vi "3.2 resolve.vi"() -> ()   [LabVIEW 2017]
panel:
  out "Numeric":i32
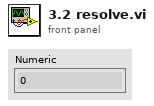
[diagram p1: front panel]
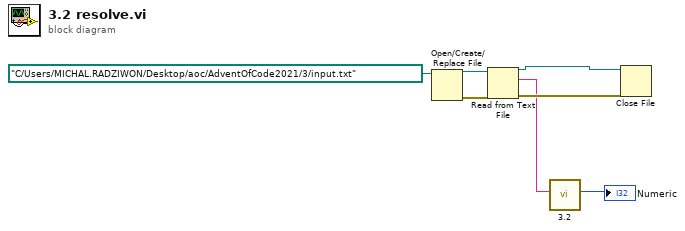
[diagram p0: block diagram]
diagram:
  n1 = Open/Create/Replace File(file path (use dialog)=path "C:/Users/MICHAL.RADZIWON/Desktop/aoc/AdventOfCode2021/3/input.txt") -> (refnum out=w5:refnum<file>, error out=w6:errorcluster)  [unwired: 5 in, 1 out]
  n2 = Read from Text File(file (use dialog)=w5, error in=w6) -> (refnum out=w4:refnum<file>, text=w2:string, error out=w3:errorcluster)  [unwired: 2 in, 1 out]
  n3 = call "3.2.vi"("String"=w2) -> ("Numeric"=→"Numeric":i32)  [unwired: 9 in, 1 out]
  n4 = Close File(refnum=w4, error in=w3) -> ()  [unwired: 2 out]
